vi "总磷总氮通讯.vi"() -> ()   [LabVIEW 2016, in "斯坦道总磷.lvlib"]
uses:
  <vilib>/Utility/config.llb/Write Key (Boolean).vi
  <vilib>/Utility/config.llb/Write Key (String).vi
  <vilib>/Plasmionique/MB Master/MB_Master/MB_Master.lvclass
  <vilib>/Utility/config.llb/NI_LVConfig.lvlib
  <vilib>/Plasmionique/MB Master/MB Master.lvlib
  <vilib>/ptbypt/NI_PtbyPt.lvlib
panel:
  out "氨氮状态告警区":u16[](array[numeric])
  out "氨氮测量数据区":u16[](array[numeric])
  out "COD测量数据区":u16[](array[numeric])
  out "COD状态告警区":u16[](array[numeric])
  out "总氮测量数据区":u16[](array[numeric])
  out "总氮状态告警区":u16[](array[numeric])
  out "总磷状态告警区":u16[](array[numeric])
  out "总磷测量数据区":u16[](array[numeric])
  out "序列号":string
  out "状态告警区":T1 {"告警代码" items=["无告警", "缺试剂告警", "缺水样告警", "缺蒸馏水告警", "缺标液告警", "仪表漏液告警", "标定异常告警", "超量程告警", "加热异常", "低试剂预警", "超上限告警", "超下限告警", "仪表内部其他异常", "滴定异常告警", "电极异常告警", "量程切换告警", "参数设置告警", "PH电极电位异常", "电导率电极异常", "浊度光度异常", "溶解氧电极异常", "溶解氧光强异常", "温度异常告警", "PH异常告警", "溶解氧异常告警", "电导率异常告警", "浊度异常告警", "叶绿素异常告警", "藻密度异常告警", "蓝绿藻异常告警", "ORP异常告警", "氨氮异常告警", "清洁刷异常告警", "SD卡异常告警", "蓝牙异常告警", "Wifi异常告警", "流程异常告警"]; "故障代码" items=["无故障", "电机故障", "温度故障", "通讯故障", "滴定故障"]}
  out "测量数据区":T2 {"单位" items=["ug/L", "mg/L", "ppm", "mg/m3", "cm", "ppb", "ug/m3", "%", "nmol/mol", "umol/mol", "MPN/L", "MPN/100ml", "ng/m3", "NTU", "无量纲", "ms/cm", "us/cm", "℃", "mV", "万个/L"]}
  out "status":bool
  out "关键参数区":T3
  in  "读关键参数区":bool
  in  "读状态告警区":bool
  in  "读测量数据区":bool
  in  "站号":u16(ring) items=["总磷"=1, "氨氮"=3]
  in  "停止":bool
  in  "启动":bool
  in  "控制命令":u16(ring) items=["启动测量"=1, "标样核查"=2, "零点核查"=3, "跨度核查"=4, "空白测试"=5, "平行样测试"=6, "加标回收"=7, "空白校准"=8, "标样校准"=9, "初始化（清洗）"=10, "停止测试"=11, "仪器重启"=12, "校时"=13, "模式设置"=14, "测量间隔设置"=15]
  in  "控制命令参数":u16[](array[numeric]) format="%04xH"
  in  "VISA Resource":refnum<visa-resource-name>
  in  "启用模块":bool
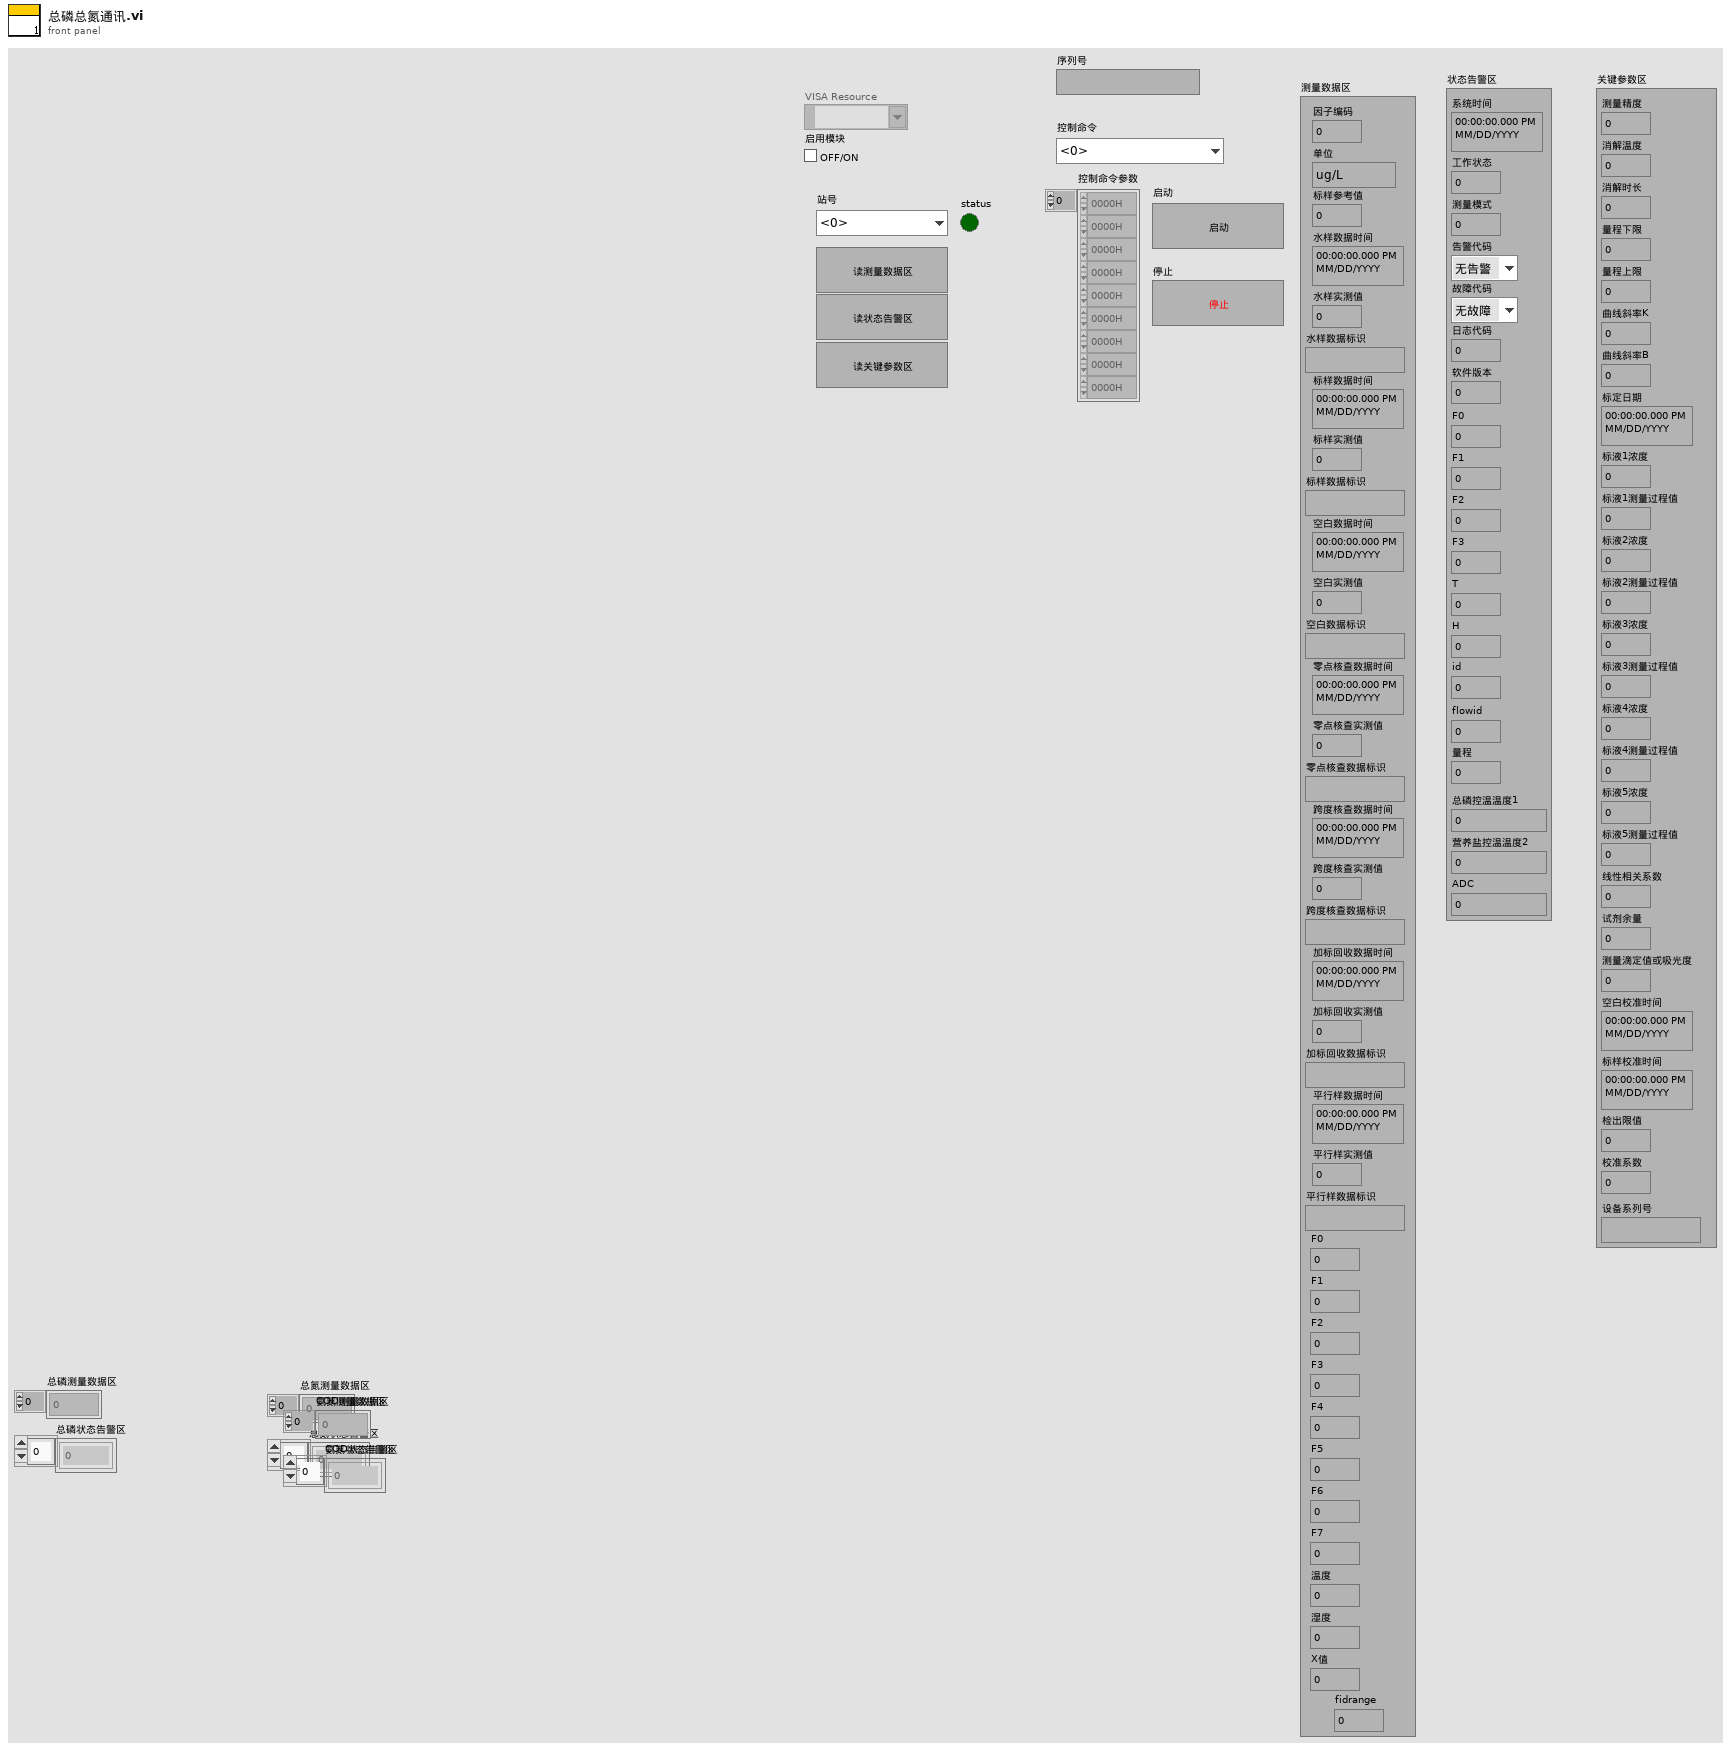
[diagram p1: front panel]
types:
  T1 = cluster{"系统时间":timestamp, "工作状态":u16, "测量模式":u16, "告警代码":u16, "故障代码":u16, "日志代码":u16, "软件版本":u16, "F0":sgl, "F1":sgl, "F2":sgl, "F3":sgl, "T":sgl, "H":sgl, "id":u16, "flowid":u16, "量程":u16, "总磷控温温度1":sgl, "营养盐控温温度2":sgl, "ADC":sgl}
  T2 = cluster{"因子编码":u32, "单位":u16, "标样参考值":sgl, "水样数据时间":timestamp, "水样实测值":sgl, "水样数据标识":string, "标样数据时间":timestamp, "标样实测值":sgl, "标样数据标识":string, "空白数据时间":timestamp, "空白实测值":sgl, "空白数据标识":string, "零点核查数据时间":timestamp, "零点核查实测值":sgl, "零点核查数据标识":string, "跨度核查数据时间":timestamp, "跨度核查实测值":sgl, "跨度核查数据标识":string, "加标回收数据时间":timestamp, "加标回收实测值":sgl, "加标回收数据标识":string, "平行样数据时间":timestamp, "平行样实测值":sgl, "平行样数据标识":string, "F0":sgl, "F1":sgl, "F2":sgl, "F3":sgl, "F4":sgl, "F5":sgl, "F6":sgl, "F7":sgl, "温度":sgl, "湿度":sgl, "X值":sgl, "fidrange":u16}
  T3 = cluster{"测量精度":u16, "消解温度":u16, "消解时长":u16, "量程下限":sgl, "量程上限":sgl, "曲线斜率K":sgl, "曲线斜率B":sgl, "标定日期":timestamp, "标液1浓度":sgl, "标液1测量过程值":sgl, "标液2浓度":sgl, "标液2测量过程值":sgl, "标液3浓度":sgl, "标液3测量过程值":sgl, "标液4浓度":sgl, "标液4测量过程值":sgl, "标液5浓度":sgl, "标液5测量过程值":sgl, "线性相关系数":sgl, "试剂余量":u32, "测量滴定值或吸光度":sgl, "空白校准时间":timestamp, "标样校准时间":timestamp, "检出限值":sgl, "校准系数":sgl, "设备系列号":string}
  T4 = typedef "NI_LVConfig.lvlib/Config Data RefNum.ctl" = refnum<k1>
  T5 = enum8{"Enabled", "Disabled", "Disabled and Grayed Out"}
  T6 = cluster{"时间标识":timestamp, "设备":string, "日志信息":string, "备注":string}
  T7 = cluster{"COD":bool, "氨氮":bool, "总氮":bool, "总磷":bool}
  T8 = cluster{"系统时间":timestamp, "工作状态":enum16{"空闲", "水样测试", "标样核查", "零点核查", "跨度核查", "空白测试", "平行样测试", "加标回收", "空白校准", "标样校准", "初始化（清洗）"}, "测量模式":enum16{"待机", "连续模式", "周期模式", "定点模式", "受控模式", "手动模式"}, "告警代码":u16, "故障代码":u16, "日志代码":u16, "软件版本":u16, "F0":sgl, "F1":sgl, "F2":sgl, "F3":sgl, "T":sgl, "H":sgl, "id":u16, "flowid":u16, "量程":u16, "总磷控温温度1":sgl, "营养盐控温温度2":sgl, "ADC":sgl}
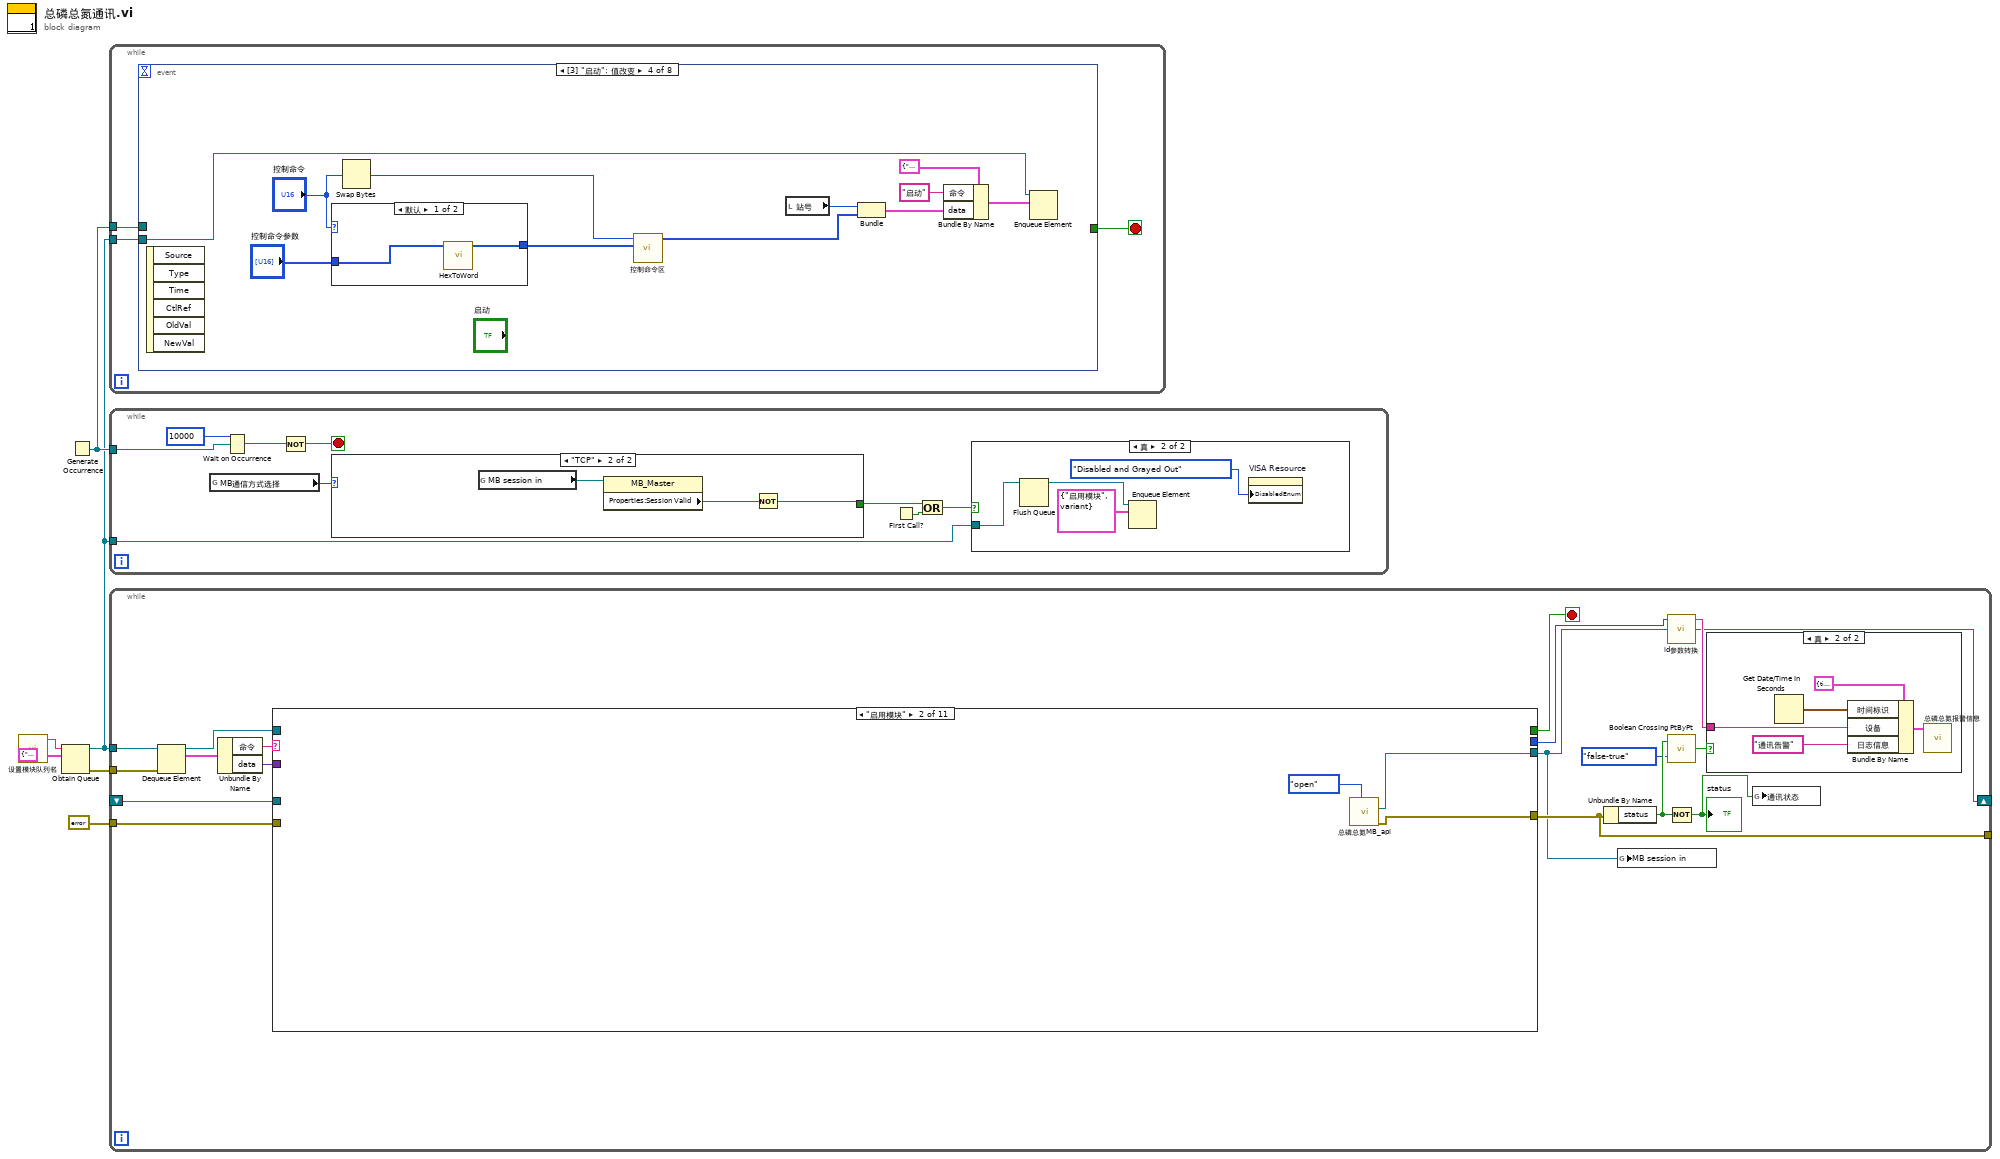
[diagram p0: block diagram]
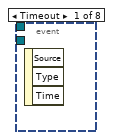
[diagram p4: hidden frame]
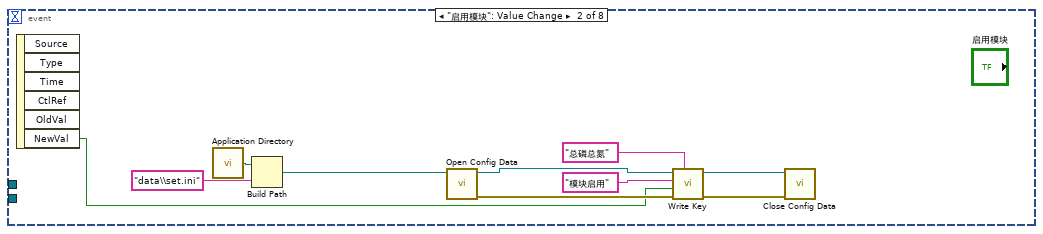
[diagram p5: hidden frame]
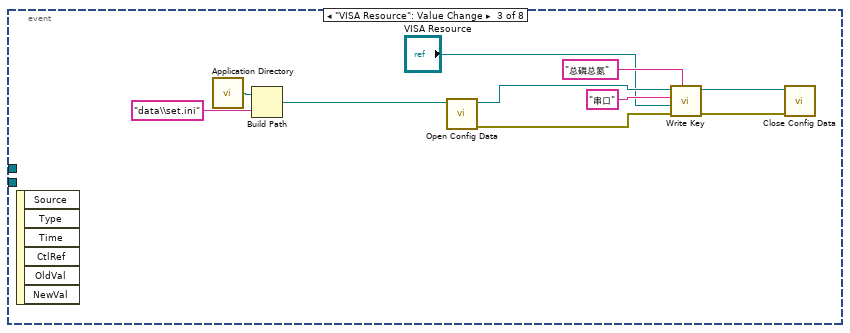
[diagram p6: hidden frame]
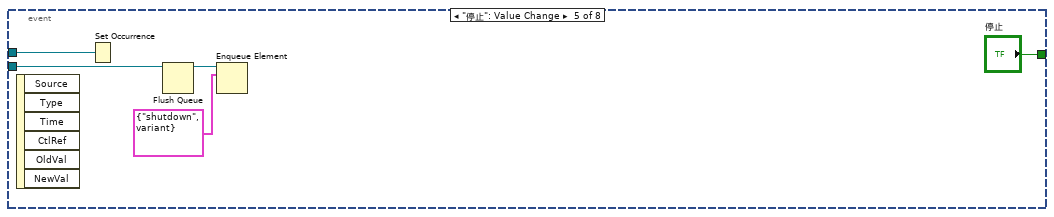
[diagram p8: hidden frame]
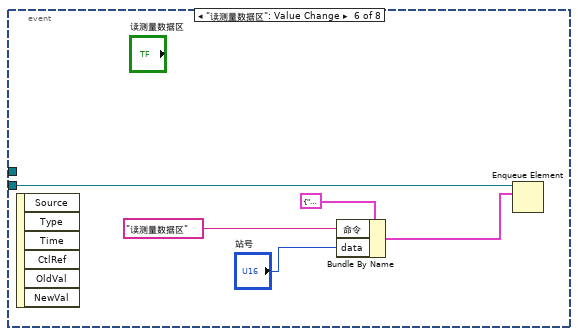
[diagram p9: hidden frame]
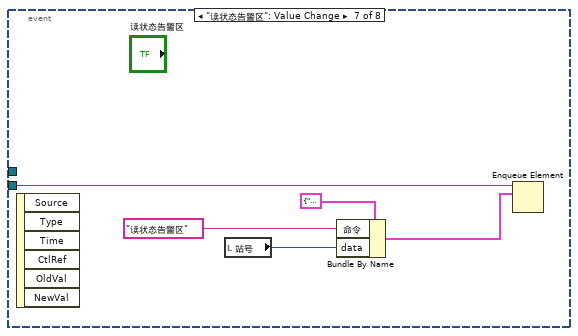
[diagram p10: hidden frame]
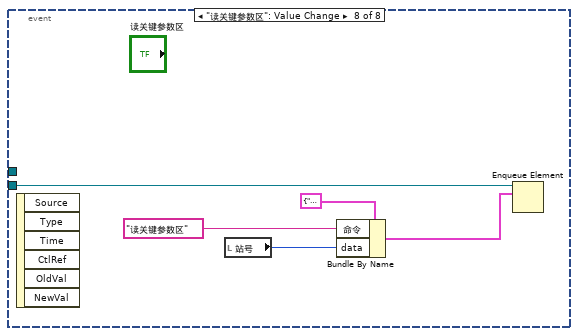
[diagram p11: hidden frame]
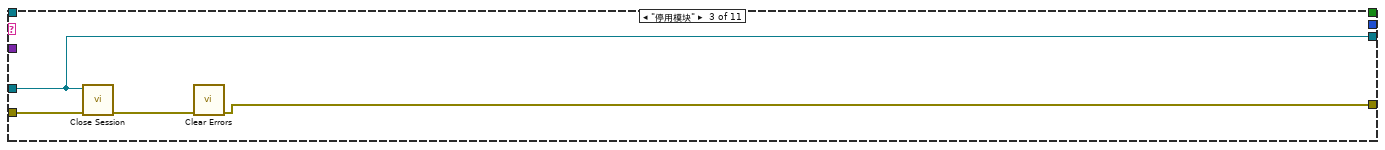
[diagram p14: hidden frame]
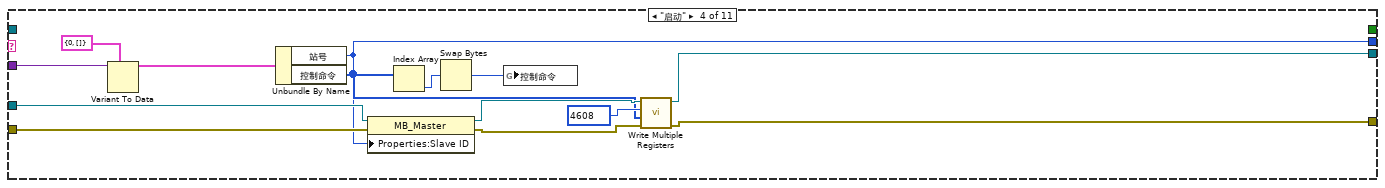
[diagram p15: hidden frame]
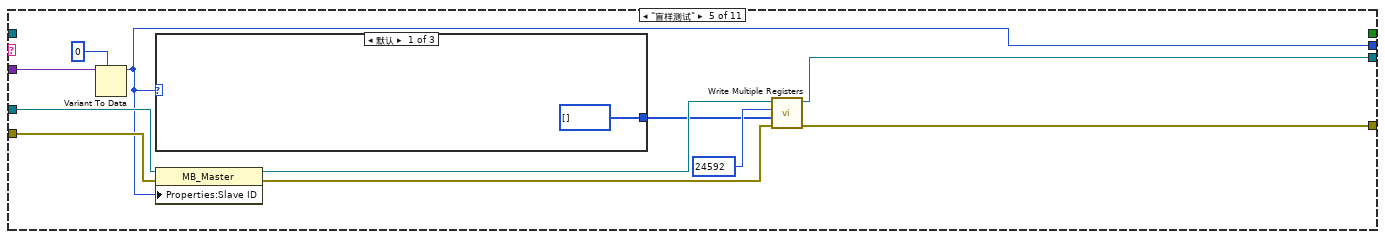
[diagram p16: hidden frame]
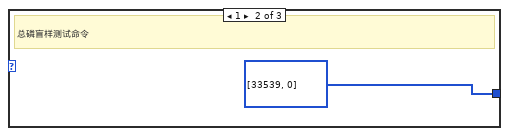
[diagram p17: hidden frame]
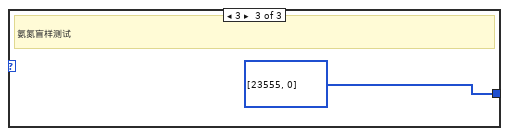
[diagram p18: hidden frame]
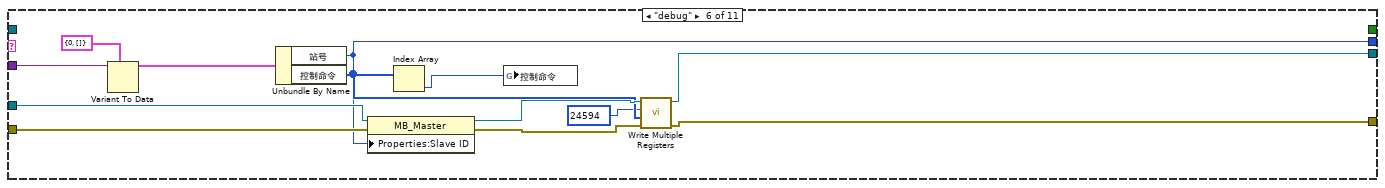
[diagram p19: hidden frame]
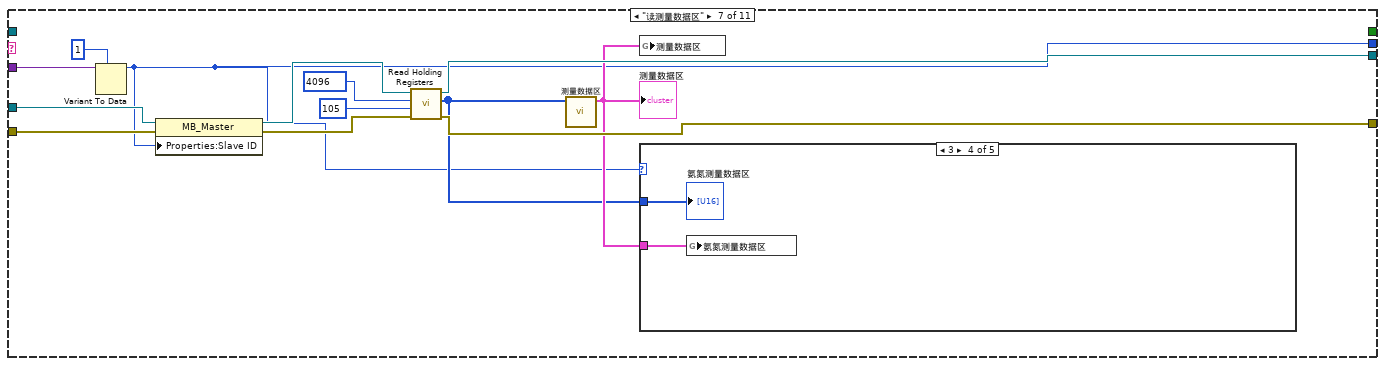
[diagram p20: hidden frame]
diagram:
  n1 = call "设置模块队列名.vi"() -> ("Msg"=w1:string)  [unwired: 5 in]
  n2 = Obtain Queue(name (unnamed)=w1, element data type=cluster{"命令":string, "data":variant} {"命令"="", "data"=variant}) -> (queue out=w2:refnum<queue>, error out=w5:errorcluster)  [unwired: 3 in, 1 out]
  n3 = Generate Occurrence() -> (w3:refnum<k4>)
  n4 = while {
    tunnel: w2 -> [w9]
    tunnel: w3 -> [w7]
    stop <- w8 stop-if-true
    n5 = event shown="[3] \"启动\": 值改变" {
      selector: _ -> [_ _ _ _ _ _ _ _]
      dyn-events: _ -> [_ _ _ _ _ _ _ _]
      timeout: _ -> [_ _ _ _ _ _ _ _]
      tunnel: w9 -> [_ _ _ w40 w47 w53 w58 w63]
      tunnel: [_ _ _ _ "停止" _ _ _] -> w8
      tunnel: w7 -> [_ _ _ _ w44 _ _ _]
      event Timeout {
        n6 = event-data() -> ()  [unwired: 1 in, 3 out]
      }
      event "启用模块": Value Change {
        n7 = event-data() -> ("NewVal"=w10:bool)  [unwired: 1 in, 5 out]
        n8 = call <vilib>:"Application Directory.vi"() -> ("Application Directory"=w12:path)
        n9 = Build Path(base path=w12, name or relative path="data\\set.ini" ("名称或相对路径")) -> (appended path=w13:path)
        n10 = call <vilib>:"Open Config Data.vi"("configuration file path"=w13) -> ("error out"=w19:errorcluster, "refnum"=w18:T4)  [unwired: 8 in, 1 out]
        n11 = call-poly <vilib>:"Write Key.vi"("section"="总磷总氮", "error in (no error)"=w19, "value"=w10, "key"="模块启用", "refnum"=w18) -> ("error out"=w15:errorcluster, "refnum out"=w11:T4)  [unwired: 4 in, 1 out]
        n12 = call <vilib>:"Close Config Data.vi"("error in (no error)"=w15, "refnum"=w11) -> ()  [unwired: 8 in, 2 out]
      }
      event "VISA Resource": Value Change {
        n13 = event-data() -> ()  [unwired: 1 in, 6 out]
        n14 = call <vilib>:"Application Directory.vi"() -> ("Application Directory"=w22:path)
        n15 = Build Path(base path=w22, name or relative path="data\\set.ini" ("名称或相对路径")) -> (appended path=w23:path)
        n16 = call <vilib>:"Open Config Data.vi"("configuration file path"=w23) -> ("error out"=w29:errorcluster, "refnum"=w28:T4)  [unwired: 8 in, 1 out]
        n17 = call-poly <vilib>:"Write Key.vi"("section"="总磷总氮", "error in (no error)"=w29, "value"="VISA Resource", "key"="串口", "refnum"=w28) -> ("error out"=w25:errorcluster, "refnum out"=w21:T4)  [unwired: 4 in, 1 out]
        n18 = call <vilib>:"Close Config Data.vi"("error in (no error)"=w25, "refnum"=w21) -> ()  [unwired: 8 in, 2 out]
      }
      event "启动": Value Change {
        n19 = event-data() -> ()  [unwired: 1 in, 6 out]
        n20 = case shown="默认" "控制命令" {
          tunnel: "控制命令参数" -> [w42 w43]
          tunnel: [w41 w43] -> w30
          frame Default {
            n21 = call "HexToWord.vi"("数组"=w42) -> ("WORD"=w41:u16[])  [unwired: 10 in]
          }
          frame 13 {
          }
        }
        n22 = Swap Bytes(anything="控制命令") -> (byte swapped=w33:u16)
        n23 = call "控制命令区.vi"("控制命令参数"=w30, "控制命令"=w33) -> ("控制命令"=w36:u16[])  [unwired: 9 in]
        n24 = local read "站号"() -> (w35:u16)
        n25 = Bundle("站号"=w35, "控制命令"=w36) -> (w34:cluster{"站号":u16, "控制命令":u16[]})  [unwired: 1 in]
        n26 = Bundle By Name(cluster=cluster{"命令":string, "data":variant} {"命令"="", "data"=variant} ("元素"), "命令"="启动", "data"=w34) -> (w38:cluster{"命令":string, "data":variant})
        n27 = Enqueue Element(queue=w40, element=w38) -> ()  [unwired: 2 in, 3 out]
      }
      event "停止": Value Change {
        n28 = event-data() -> ()  [unwired: 1 in, 6 out]
        n29 = Set Occurrence(w44) -> ()
        n30 = Flush Queue(queue=w47) -> (queue out=w46:refnum<queue>)  [unwired: 1 in, 2 out]
        n31 = Enqueue Element(queue=w46, element=cluster{"命令":string, "data":variant} {"命令"="shutdown", "data"=variant} ("元素")) -> ()  [unwired: 2 in, 3 out]
      }
      event "读测量数据区": Value Change {
        n32 = event-data() -> ()  [unwired: 1 in, 6 out]
        n33 = Bundle By Name(cluster=cluster{"命令":string, "data":variant} {"命令"="", "data"=variant} ("元素"), "命令"="读测量数据区", "data"="站号") -> (w51:cluster{"命令":string, "data":variant})
        n34 = Enqueue Element(queue=w53, element=w51) -> ()  [unwired: 2 in, 3 out]
      }
      event "读状态告警区": Value Change {
        n35 = event-data() -> ()  [unwired: 1 in, 6 out]
        n36 = local read "站号"() -> (w54:u16)
        n37 = Bundle By Name(cluster=cluster{"命令":string, "data":variant} {"命令"="", "data"=variant} ("元素"), "命令"="读状态告警区", "data"=w54) -> (w56:cluster{"命令":string, "data":variant})
        n38 = Enqueue Element(queue=w58, element=w56) -> ()  [unwired: 2 in, 3 out]
      }
      event "读关键参数区": Value Change {
        n39 = event-data() -> ()  [unwired: 1 in, 6 out]
        n40 = local read "站号"() -> (w59:u16)
        n41 = Bundle By Name(cluster=cluster{"命令":string, "data":variant} {"命令"="", "data"=variant} ("元素"), "命令"="读关键参数区", "data"=w59) -> (w61:cluster{"命令":string, "data":variant})
        n42 = Enqueue Element(queue=w63, element=w61) -> ()  [unwired: 2 in, 3 out]
      }
    }
  }
  n43 = while {
    tunnel: w3 -> [w72]
    tunnel: w2 -> [w68]
    stop <- w69 stop-if-true
    n44 = global read "总磷总氮断电保存全局变量.vi" "MB通信方式选择"() -> (w67:enum16{"串口", "TCP"})
    n45 = Wait on Occurrence(2:w72, 3:10000 ("毫秒超时(-1)")) -> (0:w70:bool)  [unwired: 1 in]
    n46 = Not(x=w70) -> (.not. x?=w69:bool)
    n47 = case shown="\"TCP\"" w67 {
      tunnel: [_ w73] -> w64
      frame "串口", Default {
      }
      frame "TCP" {
        n48 = global read "VAR总磷总氮全局变量.vi" "MB session in"() -> (w75:refnum<class "MB_Master.lvclass">)
        n49 = property class="MB_Master"(reference=w75) -> ("Properties:Session Valid"=w74:bool)  [unwired: 1 in, 2 out]
        n50 = Not(x=w74) -> (.not. x?=w73:bool)
      }
    }
    n51 = First Call?() -> (First Call?: T/F=w66:bool)
    n52 = Or(x=w64, y=w66) -> (x .or. y?=w65:bool)
    n53 = case shown="真" w65 {
      tunnel: w68 -> [_ w78]
      frame False {
      }
      frame True {
        n54 = Flush Queue(queue=w78) -> (queue out=w76:refnum<queue>)  [unwired: 1 in, 2 out]
        n55 = Enqueue Element(queue=w76, element=cluster{"命令":string, "data":variant} {"命令"="启用模块", "data"=variant} ("元素")) -> ()  [unwired: 2 in, 3 out]
        n56 = property on="VISA Resource" class="VISAName"("DisabledEnum"=T5."Disabled and Grayed Out" ("禁用")) -> ()  [unwired: 2 in, 2 out]
      }
    }
  }
  n57 = while {
    tunnel: w2 -> [w96]
    tunnel: w5 -> [w95]
    shift-right: [w80] -> _
    shift-left: _ -> [w93]
    tunnel: errorcluster {"status"=FALSE, "code"=0, "source"=""} ("error out") -> [w92]
    tunnel: [w88] -> _
    stop <- w94 stop-if-true
    n58 = Dequeue Element(queue=w96, error in (no error)=w95) -> (queue out=w89:refnum<queue>, element=w90:cluster{"命令":string, "data":variant})  [unwired: 1 in, 2 out]
    n59 = Unbundle By Name(w90) -> ("命令"=w91:string, "data"=w86:variant)
    n60 = case shown="\"启用模块\"" w91 {
      tunnel: w86 -> [_ _ _ w121 w132 w149 w159 w186 w207 w221 _]
      tunnel: w89 -> [_ _ _ _ _ _ _ _ _ _ w234]
      tunnel: [_ _ _ _ _ _ _ _ _ _ TRUE] -> w94
      tunnel: [w102 w104 w107 w124 w135 w151 w163 w194 w214 w228 w230] -> w80
      tunnel: [w103 w105 w108 w123 w134 w150 w164 w185 w215 w229 w231] -> w88
      tunnel: w93 -> [w102 _ w107 w120 w131 w148 w158 w189 w210 w224 w230]
      tunnel: w92 -> [w103 _ w110 w117 w128 w145 w156 w190 w211 w225 w232]
      tunnel: [_ _ _ w112 w125 w139 w152 w181 w203 w216 _] -> w81
      frame Default {
      }
      frame "启用模块" {
        n61 = call "总磷总氮MB_api.vi"("STEP"=enum16{"open", "read", "write", "close"}."open") -> ("error out"=w105:errorcluster, "MB session out"=w104:refnum<class "MB_Master.lvclass">)  [unwired: 8 in, 1 out]
      }
      frame "停用模块" {
        n62 = call-dynamic "Close Session.vi"("error in (no error)"=w110, "MB session in"=w107) -> ("error out"=w109:errorcluster)  [unwired: 9 in]
        n63 = call <vilib>:"Clear Errors.vi"("error in (no error)"=w109) -> ("error out"=w108:errorcluster)  [unwired: 5 in, 1 out]
      }
      frame "启动" {
        n64 = Variant To Data(type=cluster{"站号":u16, "控制命令":u16[]} {"站号"=0, "控制命令"=[]} ("输出簇"), Variant=w121) -> (data=w115:cluster{"站号":u16, "控制命令":u16[]})  [unwired: 1 in, 1 out]
        n65 = Unbundle By Name(w115) -> ("站号"=w112:u16, "控制命令"=w113:u16[])
        n66 = property class="MB_Master"(reference=w120, error in=w117, "Properties:Slave ID"=w112) -> (reference out=w119:refnum<class "MB_Master.lvclass">, error out=w118:errorcluster)
        n67 = Index Array(array=w113) -> (element=w114:u16)  [unwired: 1 in]
        n68 = Swap Bytes(anything=w114) -> (byte swapped=w111:u16)
        n69 = global write "VAR总磷总氮全局变量.vi" "控制命令"(w111) -> ()
        n70 = call <vilib>:"Write Multiple Registers.vi"("error in (no error)"=w118, "values"=w113, "starting address"=u16 4608, "MB session in"=w119) -> ("error out"=w123:errorcluster, "MB session out"=w124:refnum<class "MB_Master.lvclass">)  [unwired: 6 in]
      }
      frame "盲样测试" {
        n71 = Variant To Data(type=u8 0, Variant=w132) -> (data=w125:u8)  [unwired: 1 in, 1 out]
        n72 = case shown="默认" w125 {
          tunnel: [u16[] [] ("values") u16[] [33539, 0] ("values") u16[] [23555, 0] ("values")] -> w127
          frame Default {
          }
          frame 1 {
            # "总磷盲样测试命令"
          }
          frame 3 {
            # "氨氮盲样测试"
          }
        }
        n73 = property class="MB_Master"(reference=w131, error in=w128, "Properties:Slave ID"=w125) -> (reference out=w130:refnum<class "MB_Master.lvclass">, error out=w129:errorcluster)
        n74 = call <vilib>:"Write Multiple Registers.vi"("error in (no error)"=w129, "values"=w127, "starting address"=u16 24592, "MB session in"=w130) -> ("error out"=w134:errorcluster, "MB session out"=w135:refnum<class "MB_Master.lvclass">)  [unwired: 6 in]
      }
      frame "debug" {
        n75 = Variant To Data(type=cluster{"站号":u16, "控制命令":u16[]} {"站号"=0, "控制命令"=[]} ("输出簇"), Variant=w149) -> (data=w143:cluster{"站号":u16, "控制命令":u16[]})  [unwired: 1 in, 1 out]
        n76 = Unbundle By Name(w143) -> ("站号"=w139:u16, "控制命令"=w141:u16[])
        n77 = property class="MB_Master"(reference=w148, error in=w145, "Properties:Slave ID"=w139) -> (reference out=w147:refnum<class "MB_Master.lvclass">, error out=w146:errorcluster)
        n78 = Index Array(array=w141) -> (element=w142:u16)  [unwired: 1 in]
        n79 = global write "VAR总磷总氮全局变量.vi" "控制命令"(w142) -> ()
        n80 = call <vilib>:"Write Multiple Registers.vi"("error in (no error)"=w146, "values"=w141, "starting address"=u16 24594, "MB session in"=w147) -> ("error out"=w150:errorcluster, "MB session out"=w151:refnum<class "MB_Master.lvclass">)  [unwired: 6 in]
      }
      frame "读测量数据区" {
        n81 = Variant To Data(type=u8 1 ("Slave ID"), Variant=w159) -> (data=w152:u8)  [unwired: 1 in, 1 out]
        n82 = property class="MB_Master"(reference=w158, error in=w156, "Properties:Slave ID"=w152) -> (reference out=w157:refnum<class "MB_Master.lvclass">, error out=w155:errorcluster)
        n83 = call <vilib>:"Read Holding Registers.vi"("error in (no error)"=w155, "quantity"=u16 105, "starting address"=u16 4096, "MB session in"=w157) -> ("error out"=w164:errorcluster, "Registers"=w153:u16[], "MB session out"=w163:refnum<class "MB_Master.lvclass">)  [unwired: 5 in]
        n84 = call "测量数据区.vi"("数组"=w153) -> ("测量数据区"=w154:T2)  [unwired: 10 in]
        "测量数据区" <- w154
        n85 = global write "VAR总磷总氮全局变量.vi" "测量数据区"(w154) -> ()
        n86 = case shown="3" w152 {
          tunnel: w154 -> [_ w167 w176 w178 w180]
          tunnel: w153 -> [_ w168 w175 w177 w179]
          frame 0, Default {
          }
          frame 1 {
            n87 = global read "总磷总氮断电保存全局变量.vi" "启动参数"() -> (w166:T7)
            n88 = Unbundle By Name(w166) -> ("总氮"=w165:bool)
            n89 = case shown="真" w165 {
              tunnel: [w170 w173] -> w169
              tunnel: w167 -> [w170 w171]
              frame False {
              }
              frame True {
                # "启动总氮时间自动对齐"
                n90 = global read "VAR总磷总氮全局变量.vi" "总磷测量数据区"() -> (w172:T2)
                n91 = global read "VAR总磷总氮全局变量.vi" "总氮测量数据区"() -> (w174:T2)
                n92 = call "总磷数据时间处理.vi"("总磷修正数据输入"=w172, "总氮原始数据"=w174, "总磷原始数据"=w171) -> ("总磷修正数据输出"=w173:T2)  [unwired: 8 in]
              }
            }
            n93 = global write "VAR总磷总氮全局变量.vi" "总磷测量数据区"(w169) -> ()
            "总磷测量数据区" <- w168
          }
          frame 2 {
            n94 = global write "VAR总磷总氮全局变量.vi" "总氮测量数据区"(w176) -> ()
            "总氮测量数据区" <- w175
          }
          frame 3 {
            n95 = global write "VAR总磷总氮全局变量.vi" "氨氮测量数据区"(w178) -> ()
            "氨氮测量数据区" <- w177
          }
          frame 22 {
            n96 = global write "VAR总磷总氮全局变量.vi" "COD测量数据区"(w180) -> ()
            "COD测量数据区" <- w179
          }
        }
      }
      frame "读状态告警区" {
        n97 = Variant To Data(type=u8 1 ("Slave ID"), Variant=w186) -> (data=w181:u8)  [unwired: 1 in, 1 out]
        n98 = property class="MB_Master"(reference=w189, error in=w190, "Properties:Slave ID"=w181) -> (reference out=w188:refnum<class "MB_Master.lvclass">, error out=w187:errorcluster)
        n99 = call <vilib>:"Read Holding Registers.vi"("error in (no error)"=w187, "quantity"=u16 29, "starting address"=u16 4224, "MB session in"=w188) -> ("error out"=w185:errorcluster, "Registers"=w182:u16[], "MB session out"=w194:refnum<class "MB_Master.lvclass">)  [unwired: 5 in]
        n100 = call "状态告警区.vi"("数组"=w182) -> ("状态告警区"=w183:T8)  [unwired: 10 in]
        "状态告警区" <- w183
        n101 = Unbundle By Name(w183) -> ("id"=w184:u16)
        n102 = global write "VAR总磷总氮全局变量.vi" "状态告警区"(w183) -> ()
        n103 = case shown="3" w184 {
          tunnel: w183 -> [_ w196 w198 w200 w202]
          tunnel: w182 -> [_ w195 w197 w199 w201]
          frame 0, Default {
          }
          frame 1, 131 {
            n104 = global write "VAR总磷总氮全局变量.vi" "总磷状态告警区"(w196) -> ()
            "总磷状态告警区" <- w195
          }
          frame 2, 76 {
            n105 = global write "VAR总磷总氮全局变量.vi" "总氮状态告警区"(w198) -> ()
            "总氮状态告警区" <- w197
          }
          frame 3 {
            n106 = global write "VAR总磷总氮全局变量.vi" "氨氮状态告警区"(w200) -> ()
            "氨氮状态告警区" <- w199
          }
          frame 22 {
            n107 = global write "VAR总磷总氮全局变量.vi" "COD状态告警区"(w202) -> ()
            "COD状态告警区" <- w201
          }
        }
      }
      frame "读关键参数区" {
        n108 = Variant To Data(type=u8 1 ("Slave ID"), Variant=w207) -> (data=w203:u8)  [unwired: 1 in, 1 out]
        n109 = property class="MB_Master"(reference=w210, error in=w211, "Properties:Slave ID"=w203) -> (reference out=w209:refnum<class "MB_Master.lvclass">, error out=w208:errorcluster)
        n110 = call <vilib>:"Read Holding Registers.vi"("error in (no error)"=w208, "quantity"=u16 19, "starting address"=u16 4256, "MB session in"=w209) -> ("error out"=w215:errorcluster, "Registers"=w205:u16[], "MB session out"=w214:refnum<class "MB_Master.lvclass">)  [unwired: 5 in]
        n111 = call "关键参数区.vi"("数组"=w205) -> ("关键参数区"=w204:T3)  [unwired: 10 in]
        "关键参数区" <- w204
        n112 = global write "VAR总磷总氮全局变量.vi" "关键参数区"(w204) -> ()
      }
      frame "读序列号" {
        n113 = Variant To Data(type=u8 1 ("Slave ID"), Variant=w221) -> (data=w216:u8)  [unwired: 1 in, 1 out]
        n114 = property class="MB_Master"(reference=w224, error in=w225, "Properties:Slave ID"=w216) -> (reference out=w223:refnum<class "MB_Master.lvclass">, error out=w222:errorcluster)
        n115 = call <vilib>:"Read Holding Registers.vi"("error in (no error)"=w222, "quantity"=u16 6, "starting address"=u16 4, "MB session in"=w223) -> ("error out"=w229:errorcluster, "Registers"=w219:u16[], "MB session out"=w228:refnum<class "MB_Master.lvclass">)  [unwired: 5 in]
        n116 = call "HexToString.vi"("数组"=w219) -> ("STRING"=w218:string[])  [unwired: 10 in]
        n117 = Index Array(array=w218) -> (element=w217:string)  [unwired: 1 in]
        "序列号" <- w217
        n118 = global write "VAR总磷总氮全局变量.vi" "序列号"(w217) -> ()
      }
      frame "shutdown" {
        n119 = call-dynamic "Close Session.vi"("error in (no error)"=w232, "MB session in"=w230) -> ("error out"=w231:errorcluster)  [unwired: 9 in]
        n120 = Flush Queue(queue=w234) -> (queue out=w233:refnum<queue>)  [unwired: 1 in, 2 out]
        n121 = Release Queue(queue=w233) -> ()  [unwired: 2 in, 3 out]
      }
    }
    n122 = Unbundle By Name(w88) -> ("status"=w84:bool)
    n123 = global write "VAR总磷总氮全局变量.vi" "MB session in"(w80) -> ()
    n124 = call "id参数转换.vi"("id"=w81) -> ("table输出"=w85:string)  [unwired: 10 in]
    n125 = call <vilib>:"Boolean Crossing PtByPt.vi"("direction"=enum16{"either", "false-true", "true-false"}."false-true", "input"=w84) -> ("crossing"=w83:bool)  [unwired: 1 in]
    n126 = Not(x=w84) -> (.not. x?=w87:bool)
    "status" <- w87
    n127 = case shown="真" w83 {
      tunnel: w85 -> [_ w100]
      frame False {
      }
      frame True {
        n128 = Get Date/Time In Seconds() -> (seconds since 1Jan1904=w99:timestamp)
        n129 = Bundle By Name(cluster=T6 {"时间标识"=timestamp(0 s since 1904-01-01), "设备"="", "日志信息"="", "备注"=""} ("data in"), "时间标识"=w99, "设备"=w100, "日志信息"="通讯告警") -> (w98:T6)
        n130 = call "总磷总氮报警信息.vi"("data in"=w98) -> ()  [unwired: 10 in, 1 out]
      }
    }
    n131 = global write "VAR总磷总氮全局变量.vi" "通讯状态"(w87) -> ()
  }
